vi "main3.vi"() -> ()   [LabVIEW 2020]
panel:
  in  "String 2":string
  out "String":string
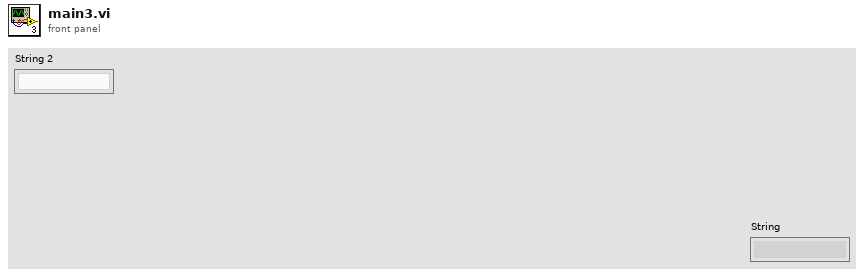
[diagram p1: front panel]
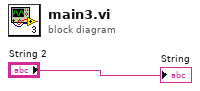
[diagram p0: block diagram]
diagram:
  "String" <- "String 2"
